vi "Create FIFO FGV Queues.vi"(8 "error in (no error)":errorcluster) -> (0 "error out":errorcluster, 4 "FIFO Idx Qs":T1)   [LabVIEW 2015, in "AIT 429 Engine.lvlib"]
uses:
  AIT 429 Engine.lvlib
  RT Controls/FIFO Idx Qs.ctl
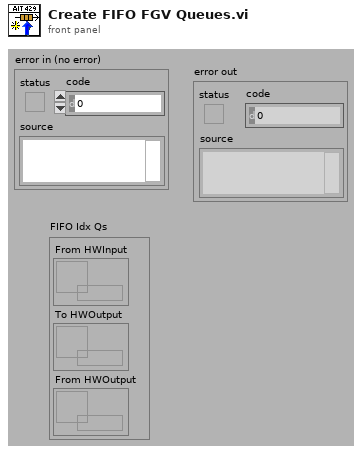
[diagram p1: front panel]
types:
  T1 = typedef "AIT 429 Engine.lvlib/FIFO Idx Qs.ctl" = cluster{"From HWInput":refnum<queue>, "To HWOutput":refnum<queue>, "From HWOutput":refnum<queue>}
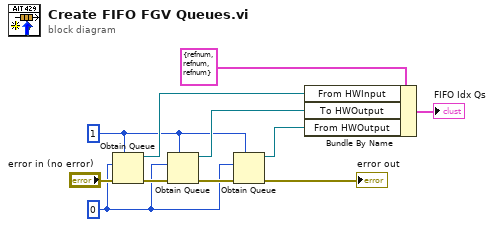
[diagram p0: block diagram]
diagram:
  w3 = 1 ("max queue size (-1, unlimited)")
  w4 = 0
  n1 = Obtain Queue(max queue size (-1, unlimited)=w3, element data type=w4, error in (no error)="error in (no error)") -> (queue out=w7:refnum<queue>, error out=w10:errorcluster)  [unwired: 2 in, 1 out]
  n2 = Obtain Queue(max queue size (-1, unlimited)=w3, element data type=w4, error in (no error)=w10) -> (queue out=w6:refnum<queue>, error out=w5:errorcluster)  [unwired: 2 in, 1 out]
  n3 = Obtain Queue(max queue size (-1, unlimited)=w3, element data type=w4, error in (no error)=w5) -> (queue out=w2:refnum<queue>, error out=→"error out":errorcluster)  [unwired: 2 in, 1 out]
  n4 = Bundle By Name(cluster=T1 {"From HWInput"=refnum, "To HWOutput"=refnum, "From HWOutput"=refnum} ("FIFO Idx Qs"), "From HWInput"=w7, "To HWOutput"=w6, "From HWOutput"=w2) -> (→"FIFO Idx Qs":T1)
